vi "Interface - By List.vi"(7 "Msg Chain":string, 8 "error in (no error)":errorcluster {"code" format="Error %.0f"}, 10 "Interfaces":refnum<class "Interface Documenation.lvclass">[](array[class]), 11 "VIDoc Printer - Confluence In":refnum<class "VIDoc Printer - Confluence.lvclass">) -> (0 "error out":errorcluster {"code" format="Error %.0f"}, 3 "VIDoc Printer - Confluence Out":refnum<class "VIDoc Printer - Confluence.lvclass">)   [LabVIEW 2023, in "VIDoc Printer - Confluence.lvlib" / "VIDoc Printer - Confluence.lvclass"]
uses:
  VIDoc Printer - Confluence.lvclass
  C:/projects/DMC/Tooling/Git-Action-Service/Source/Documentation Generation/Printers/Printer/VIDoc Printer.lvclass
  Parsing/Interface Documenation/Interface Documenation.lvclass
  Confluence Formatting/Types/Format Combo Box.ctl
  Printer/VIDoc Printer.lvclass/VIDoc Printer.ctl
  VIDoc Printer - Confluence.lvclass/VIDoc Printer - Confluence.ctl
  Parsing/Interface Documenation/Interface Documenation.lvclass/Interface Documenation.ctl
  Parsing/Interface Documenation/Get Interface Info.vi
  Printer/Accessors/Get Interface Settings - List Detail Level.vi
  Accessors/Get Interface List Expand.vi
  Confluence Formatting/Confluence Formatting.lvlib
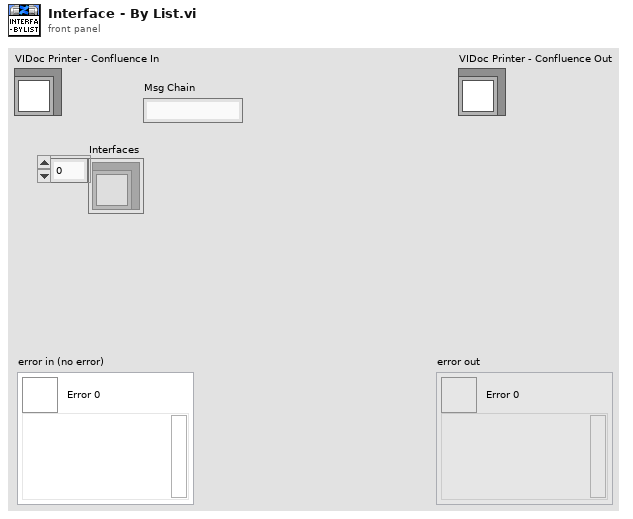
[diagram p1: front panel]
types:
  T1 = typedef "Confluence Formatting.lvlib/Format Combo Box.ctl" = string
  T2 = typedef "VIDoc Printer.lvlib/Printer Settings.lvclass/Detail Level Enum.ctl" = enum16{"None", "Minimal", "Standard", "Full"}
  T3 = typedef "VIDoc Parsing.lvlib/Base Class Info Cluster.ctl" = cluster{"Name":string, "Icon":T4, "Version":cluster{"Major":u16, "Minor":u16, "Fix":u16, "Build":u16}, "Description":string, "Friends":string[], "ChildRefsRestricted":bool, "TransferMustOverrides":bool, "Path":path, "Qualified Name":string, "Class Scope":enum32{"invalid scope", "public", "private", "protected", "community"}}
  T4 = typedef "imagedata.ctl" = cluster{"image type":i32, "image depth":i32, "image":u8[], "mask":u8[], "colors":u32[], "Rectangle":cluster{"left":i16, "top":i16, "right":i16, "bottom":i16}}
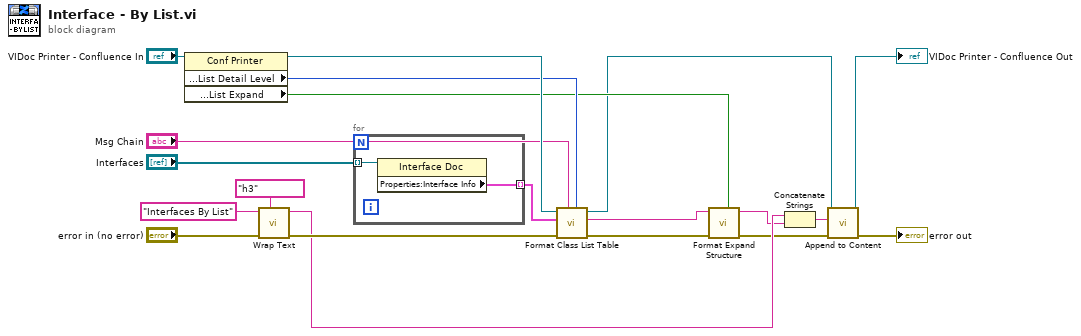
[diagram p0: block diagram]
diagram:
  n1 = property class="Conf Printer"(reference="VIDoc Printer - Confluence In") -> (reference out=w17:refnum<class "VIDoc Printer - Confluence.lvclass">, "Properties:Settings:Interfaces:List Detail Level"=w3:T2, "Properties:Expand?:Interface:List Expand"=w2:bool)  [unwired: 1 in, 1 out]
  n2 = call "Wrap Text.vi"("Formatting"=T1 "h3", "Error in"="error in (no error)", "String"="Interfaces By List") -> ("Error out"=w18:errorcluster, "Wrapped String"=w14:string)  [unwired: 7 in]
  n3 = for {
    tunnel: "Interfaces" -> [w22] mode=indexing
    tunnel: [w21] -> w4 mode=indexing
    n4 = property class="Interface Doc"(reference=w22) -> ("Properties:Interface Info"=w21:T3)  [unwired: 1 in, 2 out]
  }
  n5 = call "Format Class List Table.vi"("Detail Level"=w3, "Msg Chain in"="Msg Chain", "error in (no error)"=w18, "Class Info Array"=w4, "VIDoc Printer - Confluence In"=w17) -> ("error out"=w15:errorcluster, "Table Text"=w6:string, "VIDoc Printer - Confluence Out"=w1:refnum<class "VIDoc Printer - Confluence.lvclass">)  [unwired: 4 in]
  n6 = call "Format Expand Structure.vi"("Enable? (T)"=w2, "Error in"=w15, "Content"=w6) -> ("Error out"=w7:errorcluster, "Expand String"=w5:string)  [unwired: 7 in]
  n7 = Concatenate Strings(w14, w5) -> (w16:string)
  n8 = call "Append to Content.vi"("error in (no error)"=w7, "Content"=w16, "VIDoc Printer - Confluence In"=w1) -> ("error out"=→"error out":errorcluster, "VIDoc Printer - Confluence Out"=→"VIDoc Printer - Confluence Out":refnum<class "VIDoc Printer - Confluence.lvclass">)  [unwired: 7 in]
